vi "dvp Vi Get Gamma.vi"(10 "pGamma":i32, 11 "handle":u32) -> (2 "pGamma out":i32, 3 "function return":u32(ring))   [LabVIEW 2018, in "LabViewDVPCamera.lvlib"]
doc: "LabviewDvp2Api dvpStatus dvpViGetGamma(dvpHandle handle, dvpInt32 *pGamma);"
uses:
  LabViewDVPCamera.lvlib
  LabViewDVPCamera/LabViewDVPCamera.dll
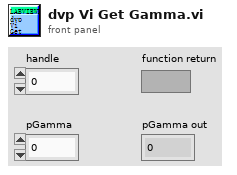
[diagram p1: front panel]
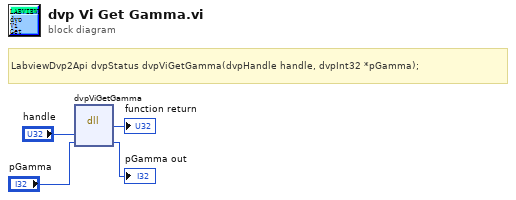
[diagram p0: block diagram]
diagram:
  # "LabviewDvp2Api dvpStatus dvpViGetGamma(dvpHandle handle, dvpInt32 *pGamma);"
  n1 = dll-call lib="C:/Program Files (x86)/DVP2 Labview cn 64/Sample/LabViewDVPCamera/LabViewDVPCamera.*" fn="dvpViGetGamma"("handle"="handle", "pGamma"="pGamma") -> (→"function return":u32, "pGamma"=→"pGamma out":i32)  [unwired: 4 in, 2 out]
